vi "Count Cargo (SubVI).vi"(5 "shooting":bool, 6 "sucking":bool, 7 "indexerVelocity":dbl, 8 "ballsShotIn":dbl, 9 "cargoSensors":T1, 10 "indexerDesired":dbl, 11 "ballsCollectedIn":dbl) -> (2 "ballsShot":dbl, 3 "ballsCollected":dbl)   [LabVIEW 2020]
uses:
  Cargo Sensors.ctl
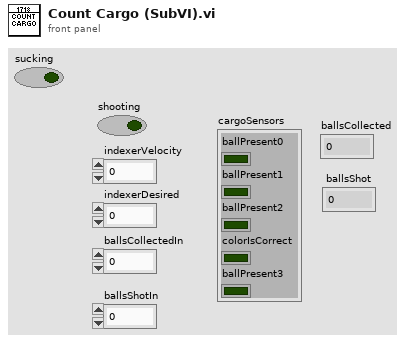
[diagram p1: front panel]
types:
  T1 = typedef "Cargo Sensors.ctl" = cluster{"ballPresent0":bool, "ballPresent1":bool, "ballPresent2":bool, "colorIsCorrect":bool, "ballPresent3":bool}
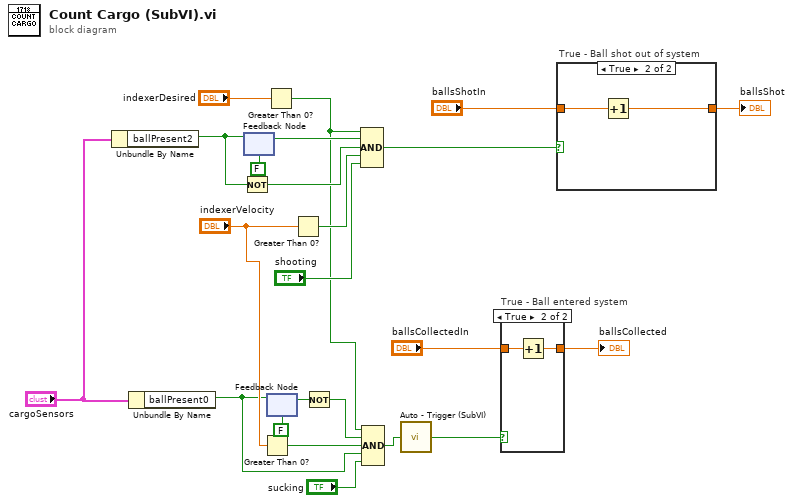
[diagram p0: block diagram]
diagram:
  n1 = Unbundle By Name("cargoSensors") -> ("ballPresent2"=w17:bool)
  n2 = Unbundle By Name("cargoSensors") -> ("ballPresent0"=w3:bool)
  n3 = Not(x=w17) -> (.not. x?=w5:bool)
  n4 = feedback #1(FALSE ("ballPresent1")) -> (w18:bool)
  n5 = feedback-in #1(w17) -> ()
  n6 = Greater Than 0?(x="indexerVelocity") -> (x > 0?=w2:bool)
  n7 = Greater Than 0?(x="indexerDesired") -> (x > 0?=w4:bool)
  n8 = feedback #2(FALSE ("ballPresent1")) -> (w7:bool)
  n9 = feedback-in #2(w3) -> ()
  n10 = Greater Than 0?(x="indexerVelocity") -> (x > 0?=w13:bool)
  n11 = Not(x=w7) -> (.not. x?=w1:bool)
  n12 = Compound Arithmetic op=AND(w4, w18, w5, w13, "shooting") -> (w9:bool)
  n13 = Compound Arithmetic op=AND(w4, w1, w2, w3, "sucking") -> (w21:bool)
  n14 = call "Auto - Trigger (SubVI).vi"("Trigger"=w21) -> ("Trigger Output"=w22:bool)
  n15 = case "True - Ball entered system" shown="True" w22 {
    tunnel: [w24 w26] -> w20
    tunnel: "ballsCollectedIn" -> [w24 w25]
    frame False {
    }
    frame True {
      n16 = Increment(x=w25) -> (x+1=w26:dbl)
    }
  }
  "ballsCollected" <- w20
  n17 = case "True - Ball shot out of system" shown="True" w9 {
    tunnel: [w27 w29] -> w15
    tunnel: "ballsShotIn" -> [w27 w28]
    frame False {
    }
    frame True {
      n18 = Increment(x=w28) -> (x+1=w29:dbl)
    }
  }
  "ballsShot" <- w15
